vi "nD Line Search.vi"(0 "J":dbl[][](array[numeric]) format="%.2f", 5 "result":dbl[][](array[numeric]) format="%.2f", 6 "list of variables":i32[](array[numeric])=[0, 0], 7 "table":i32[][][](array[numeric]), 8 "TOLX":dbl=1e-07 format="%.2e", 9 "alpha":dbl=0.0001 format="%.2e", 10 "P":dbl[](array[numeric]) format="%.2f", 11 "X":dbl[](array[numeric]) format="%.2f") -> (2 "index":u32, 3 "X (new)":dbl[](array[numeric]) format="%.2f")   [LabVIEW 2010, in "NI_Gmath.lvlib"]
uses:
  NI_Gmath.lvlib
  Real Dot Product.vi
  NI_AALBase.lvlib
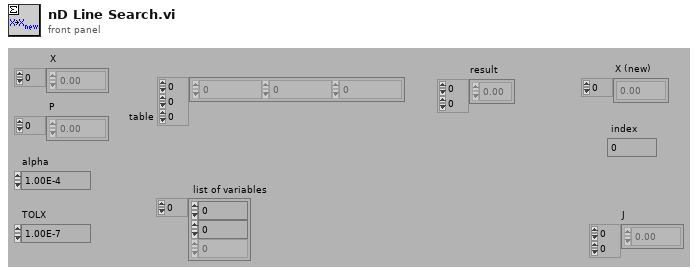
[diagram p1: front panel]
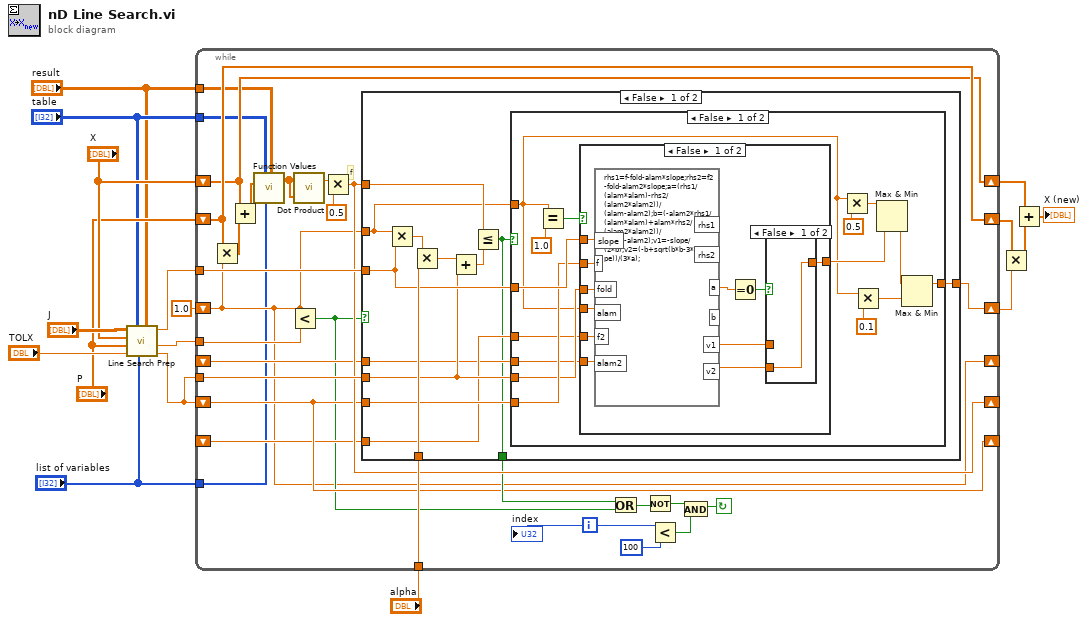
[diagram p0: block diagram]
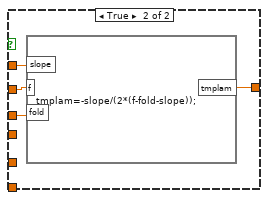
[diagram p3: hidden frame]
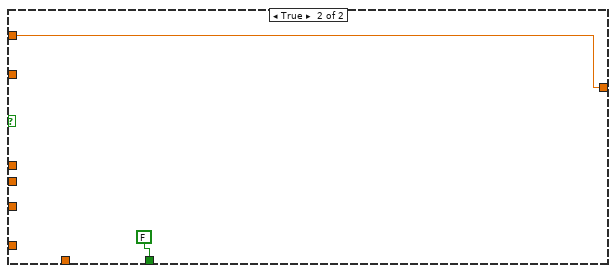
[diagram p5: hidden frame]
diagram:
  n1 = call "Line Search Prep.vi"("result"="result", "list of variables"="list of variables", "table"="table", "TOLX"="TOLX", "P"="P", "X"="X", "J"="J") -> ("F(X)*F(X)"=w12:dbl, "tolerance"=w14:dbl, "X * Y"=w13:dbl)  [unwired: 2 in]
  n2 = while {
    tunnel: w12 -> [w41]
    tunnel: w13 -> [w42]
    tunnel: "alpha" -> [w43]
    tunnel: w14 -> [w44]
    shift-left: _ -> [w34]
    shift-right: [w35] -> _
    shift-left: w12 -> [w35]
    shift-right: [w37] -> _
    shift-left: _ -> [w33]
    shift-right: [w27] -> _
    shift-left: 1.0 -> [w27]
    shift-right: [w26] -> w10
    shift-left: "P" -> [w32]
    shift-right: [w32] -> w9
    shift-left: "X" -> [w31]
    shift-right: [w31] -> w11
    tunnel: "result" -> [w20]
    tunnel: "table" -> [w19]
    tunnel: "list of variables" -> [w18]
    i -> [w30]
    stop <- w21 continue-if-true
    # "f"
    n3 = Multiply(x=w32, y=w27) -> (x*y=w45:dbl[])
    n4 = Add(x=w31, y=w45) -> (x+y=w25:dbl[])
    n5 = call "Function Values.vi"("result"=w20, "list of variables"=w18, "table"=w19, "X"=w25) -> ("F(X)"=w40:dbl[])  [unwired: 7 in]
    n6 = Less?(x=w27, y=w44) -> (x < y?=w29:bool)
    n7 = call-poly "Dot Product.vi"("Y Vector"=w40, "X Vector"=w40) -> ("X * Y"=w39:dbl)  [unwired: 1 out]
    n8 = Multiply(x=w39, y=0.5) -> (x*y=w37:dbl)
    n9 = case shown="False" w29 {
      tunnel: w43 -> [w58 _]
      tunnel: w27 -> [w53 w92]
      tunnel: w42 -> [w51 _]
      tunnel: w41 -> [w49 _]
      tunnel: w37 -> [w54 _]
      tunnel: [w46 FALSE] -> w36
      tunnel: [w52 w92] -> w26
      tunnel: w35 -> [w50 _]
      tunnel: w34 -> [w48 _]
      tunnel: w33 -> [w47 _]
      frame False {
        n10 = Multiply(x=w53, y=w51) -> (x*y=w57:dbl)
        n11 = Multiply(x=w57, y=w58) -> (x*y=w56:dbl)
        n12 = Add(x=w56, y=w49) -> (x+y=w55:dbl)
        n13 = Less Or Equal?(x=w54, y=w55) -> (x <= y?=w46:bool)
        n14 = case shown="False" w46 {
          tunnel: w53 -> [w61 w91]
          tunnel: [w65 w91] -> w52
          tunnel: w51 -> [w64 _]
          tunnel: w50 -> [w63 _]
          tunnel: w49 -> [w62 _]
          tunnel: w48 -> [w60 _]
          tunnel: w47 -> [w59 _]
          frame False {
            n15 = Equal?(x=w61, y=1.0) -> (x = y?=w72:bool)
            n16 = case shown="False" w72 {
              tunnel: [w75 w90] -> w69
              tunnel: w64 -> [w84 w89]
              tunnel: w63 -> [w83 w88]
              tunnel: w62 -> [w82 w87]
              tunnel: w61 -> [w81 _]
              tunnel: w60 -> [w80 _]
              tunnel: w59 -> [w79 _]
              frame False {
                n17 = formula code="rhs1=f-fold-alam*slope;rhs2=f2-fold-alam2*slope;a=(rhs1/(alam*alam)-rhs2/(alam2*alam2))/(alam-alam2);b=(-alam2*rhs1/(alam*alam)+alam*rhs2/(alam2*alam2))/(alam-alam2);v1=-slope/(2*b);v2=(-b+sqrt(b*b-3*a*slope))/(3*a);"("slope"=w84, "f"=w83, "fold"=w82, "alam"=w81, "f2"=w80, "alam2"=w79) -> ("a"=w78:dbl, "v1"=w76:dbl, "v2"=w74:dbl)  [unwired: 3 out]
                n18 = Equal To 0?(x=w78) -> (x = 0?=w77:bool)
                n19 = case shown="False" w77 {
                  tunnel: w76 -> [_ w86]
                  tunnel: [w85 w86] -> w75
                  tunnel: w74 -> [w85 _]
                  frame False {
                  }
                  frame True {
                  }
                }
              }
              frame True {
                n20 = formula code="tmplam=-slope/(2*(f-fold-slope));"("slope"=w89, "f"=w88, "fold"=w87) -> ("tmplam"=w90:dbl)
              }
            }
            n21 = Multiply(x=w61, y=0.5) -> (x*y=w70:dbl)
            n22 = Multiply(x=w61, y=0.1) -> (x*y=w66:dbl)
            n23 = Max & Min(x=w70, y=w69) -> (min(x,y)=w67:dbl)  [unwired: 1 out]
            n24 = Max & Min(x=w67, y=w66) -> (max(x,y)=w65:dbl)  [unwired: 1 out]
          }
          frame True {
          }
        }
      }
      frame True {
      }
    }
    n25 = Or(x=w36, y=w29) -> (x .or. y?=w28:bool)
    n26 = Not(x=w28) -> (.not. x?=w22:bool)
    n27 = Less?(x=w30, y=100) -> (x < y?=w23:bool)
    n28 = And(x=w22, y=w23) -> (x .and. y?=w21:bool)
    "index" <- w30
  }
  n29 = Multiply(x=w9, y=w10) -> (x*y=w8:dbl[])
  n30 = Add(x=w11, y=w8) -> (x+y=→"X (new)":dbl[])
